vi "SLL DE AI Driver.vi"(7 "AI Driver Option":T2, 8 "error in (no error)":errorcluster, 10 "AI Channel Name Array":T1[](array[typedef]), 11 "AI Channel Name":T1) -> (0 "error out":errorcluster, 2 "AI Channel Value Array":dbl[](array[numeric]), 3 "AI Channel Value":dbl)   [LabVIEW 2009]
doc: "Copyright © 2005, Soliton Technologies.\nAll rights reserved."
uses:
  Controls/SLL DE AI Global Options.ctl
  Controls/SLL DE List of Analog Inputs.ctl
  Controls/SLL DE DAQ Global Elements.ctl
  Controls/SLL DE DAQ Global Options.ctl
  <vilib>/DAQmx/read.llb/DAQmx Read (Analog 1D DBL 1Chan NSamp).vi
  <vilib>/Analysis/NI_AALBase.lvlib
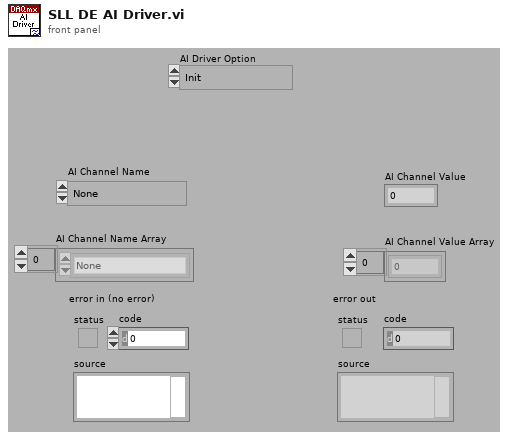
[diagram p1: front panel]
types:
  T1 = typedef "SLL DE List of Analog Inputs.ctl" = enum16{"None"}
  T2 = typedef "SLL DE AI Global Options.ctl" = enum16{"Init", "Write Line", "Write Array", "Read Line", "Read Array", "Read Full Status", "Write Full Status"}
  T3 = typedef "SLL DE DAQ Global Elements.ctl" = enum16{"AI Error", "AO Error", "DI Error", "DO Error", "AI Restart", "DI Restart", "AI Running", "AO Running", "DI Running", "DO Running", "DAQ Exit?"}
  T4 = typedef "SLL DE DAQ Global Options.ctl" = enum16{"Init", "Write 1", "Read 1", "Write Array", "Read Array", "Clear"}
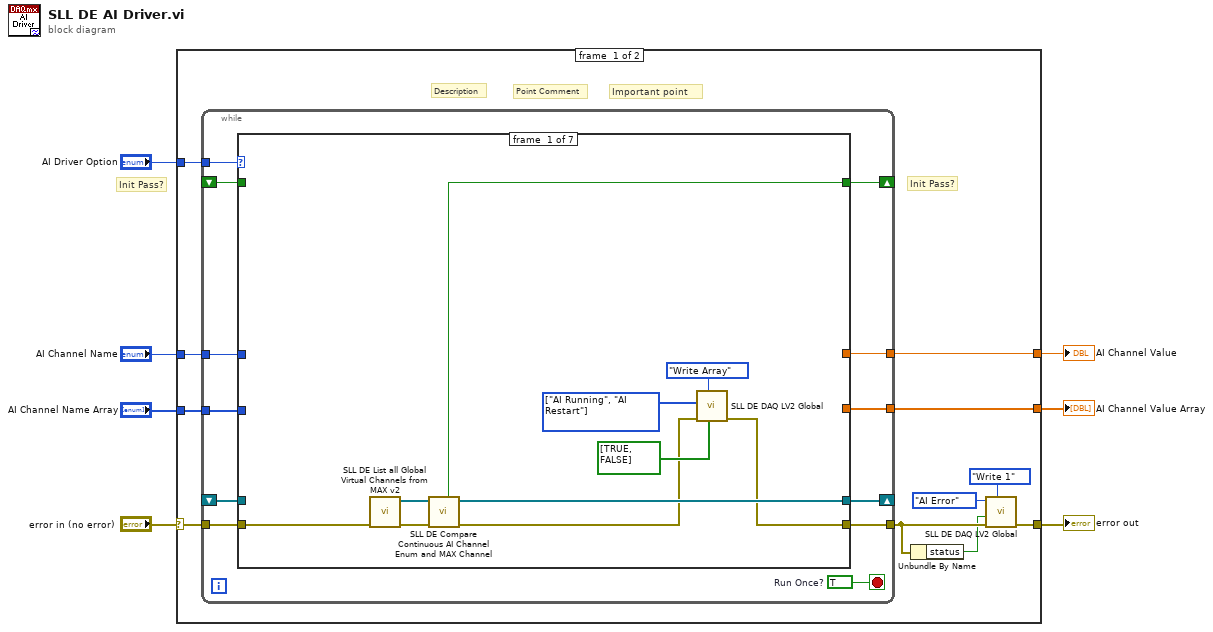
[diagram p0: block diagram]
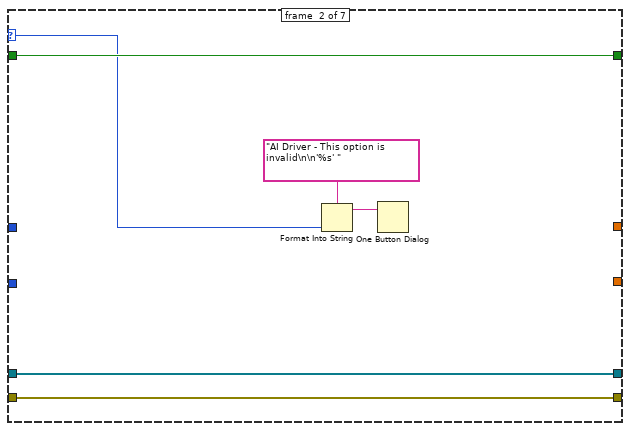
[diagram p2: hidden frame]
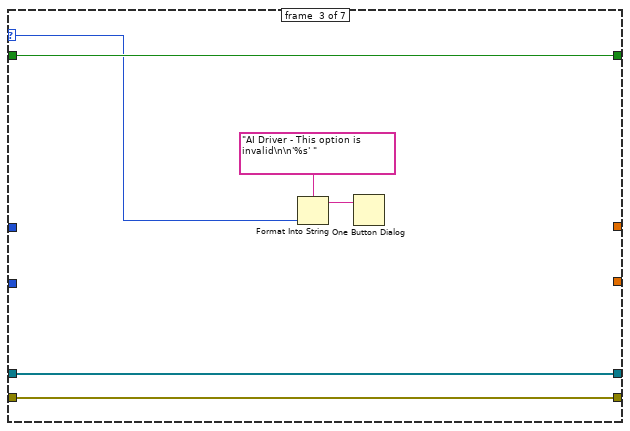
[diagram p3: hidden frame]
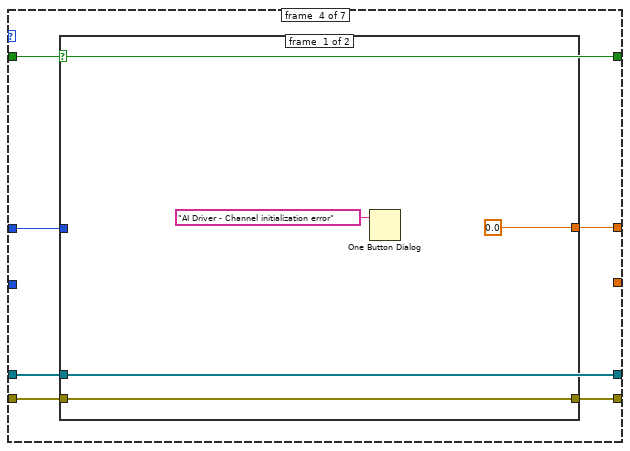
[diagram p4: hidden frame]
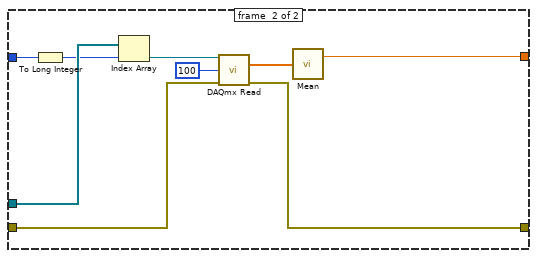
[diagram p5: hidden frame]
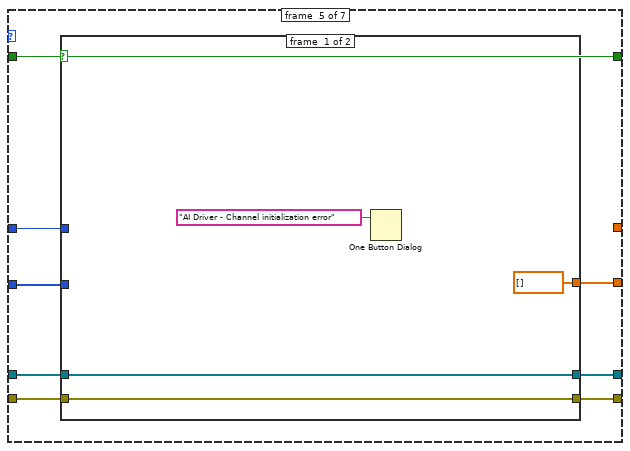
[diagram p6: hidden frame]
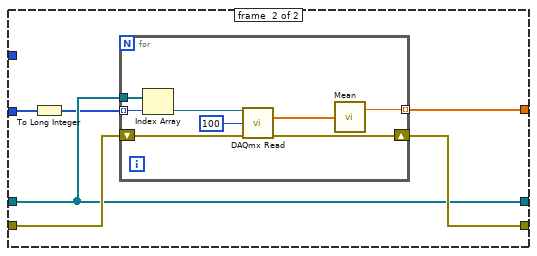
[diagram p7: hidden frame]
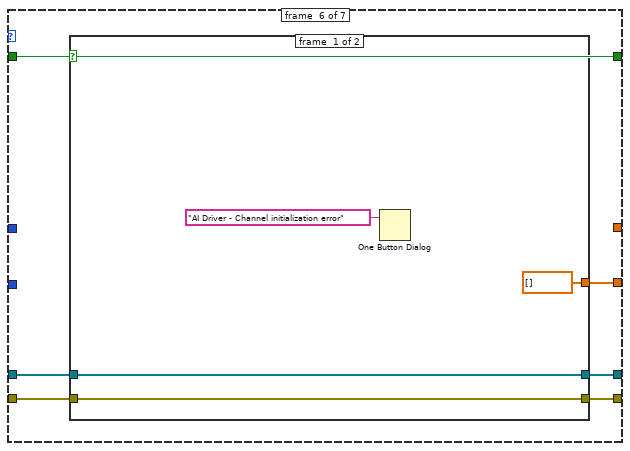
[diagram p8: hidden frame]
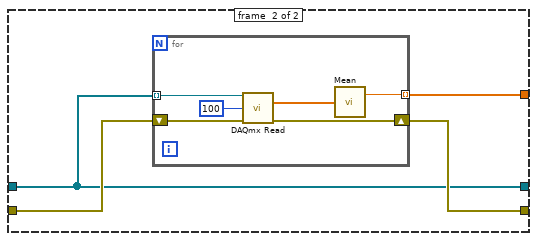
[diagram p9: hidden frame]
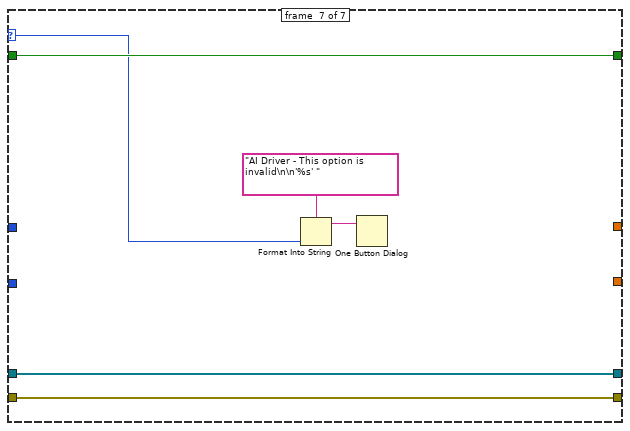
[diagram p10: hidden frame]
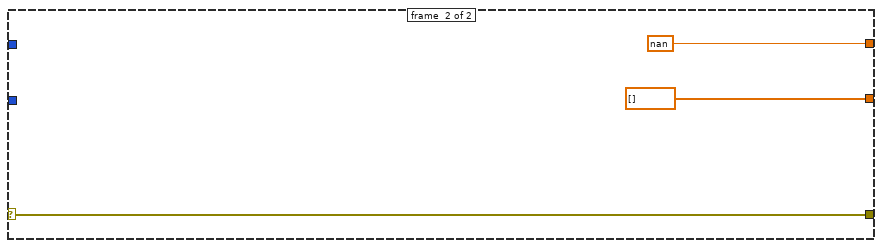
[diagram p11: hidden frame]
diagram:
  # "Init Pass?"
  n1 = case shown="No Error" "error in (no error)" {
    selector: "error in (no error)" -> [w18 w125]
    tunnel: [w11 w125] -> w6
    tunnel: "AI Driver Option" -> [w17 _]
    tunnel: "AI Channel Name" -> [w16 _]
    tunnel: [w15 nan ("mean")] -> w3
    tunnel: "AI Channel Name Array" -> [w14 _]
    tunnel: [w13 dbl[] []] -> w1
    frame #0 {
      # "Init Pass?"
      # "Point Comment"
      # "Important point"
      # "Description"
      n2 = while {
        tunnel: w18 -> [w29]
        tunnel: [w28] -> w9
        shift-right: [w27] -> _
        shift-left: _ -> [w24]
        shift-right: [w26] -> _
        shift-left: _ -> [w23]
        tunnel: w17 -> [w25]
        tunnel: w16 -> [w22]
        tunnel: [w21] -> w15
        tunnel: w14 -> [w20]
        tunnel: [w19] -> w13
        stop <- w30 stop-if-true
        w30 = TRUE  # Run Once?
        n3 = case shown="\"Read Line\"" w25 {
          selector: w25 -> [_ w41 w47 _ _ _ w117]
          tunnel: w29 -> [w38 w44 w50 w56 w78 w102 w121]
          tunnel: [w31 w44 w50 w55 w75 w98 w121] -> w28
          tunnel: [w37 w46 w52 w53 w71 w97 w122] -> w27
          tunnel: [w36 w45 w51 w58 w74 w99 w120] -> w26
          tunnel: w24 -> [_ w46 w52 w53 w71 w97 w122]
          tunnel: w23 -> [_ w45 w51 w58 w77 w101 w120]
          tunnel: w22 -> [_ _ _ w57 w76 _ _]
          tunnel: [_ _ _ w54 _ _ _] -> w21
          tunnel: w20 -> [_ _ _ _ w73 _ _]
          tunnel: [_ _ _ _ w72 w100 _] -> w19
          frame #0 {
            w34 = T3[] [enum."AI Running", enum."AI Restart"] items=["AI Error", "AO Error", "DI Error", "DO Error", "AI Restart", "DI Restart", "AI Running", "AO Running", "DI Running", "DO Running", "DAQ Exit?"] ("Elements Array")
            n4 = call "SLL DE List all Global Virtual Channels from MAX v2.vi"("error in (no error)"=w38) -> ("error out"=w39:errorcluster, "Analog Input"=w40:refnum<k21>[])  [unwired: 4 in, 5 out]
            n5 = call "SLL DE Compare Continuous AI Channel Enum and MAX Channel.vi"("error in (no error)"=w39, "Analog Input Channels"=w40) -> ("error out"=w32:errorcluster, "Channels Out"=w36:refnum<k21>[], "Pass?"=w37:bool)  [unwired: 7 in]
            n6 = call "SLL DE DAQ LV2 Global.vi"("Status Array In"=bool[] [TRUE, FALSE], "Option"=SLL_DE_DAQ_Global_Options."Write Array", "error in (no error)"=w32, "Elements Array"=w34) -> ("error out"=w31:errorcluster)  [unwired: 5 in, 2 out]
          }
          frame #1 {
            n7 = Format Into String(format string="AI Driver - This option is invalid\n\n'%s' " ("message"), w41) -> (resulting string=w42:string)  [unwired: 2 in, 1 out]
            n8 = One Button Dialog(message=w42) -> ()  [unwired: 1 in, 1 out]
          }
          frame #2 {
            n9 = Format Into String(format string="AI Driver - This option is invalid\n\n'%s' " ("message"), w47) -> (resulting string=w48:string)  [unwired: 2 in, 1 out]
            n10 = One Button Dialog(message=w48) -> ()  [unwired: 1 in, 1 out]
          }
          frame #3 {
            n11 = case shown="True" w53 {
              tunnel: w58 -> [_ w68]
              tunnel: w57 -> [_ w67]
              tunnel: w56 -> [w60 w64]
              tunnel: [w60 w63] -> w55
              tunnel: [0.0 ("mean") w62] -> w54
              frame #0 {
                n12 = One Button Dialog(message="AI Driver - Channel initialization error") -> ()  [unwired: 1 in, 1 out]
              }
              frame #1 {
                n13 = To Long Integer(number=w67) -> (32bit integer=w66:i32)
                n14 = Index Array(array=w68, index=w66) -> (element=w65:refnum<k21>)
                n15 = call-poly <vilib>:"DAQmx Read.vi"("task/channels in"=w65, "number of samples per channel"=100, "error in"=w64) -> ("data"=w69:dbl[], "error out"=w63:errorcluster)  [unwired: 10 in, 1 out]
                n16 = call <vilib>:"Mean.vi"("X"=w69) -> ("mean"=w62:dbl)  [unwired: 1 out]
              }
            }
          }
          frame #4 {
            n17 = case shown="True" w71 {
              tunnel: w77 -> [w80 w85]
              tunnel: w76 -> [_ _]
              tunnel: w78 -> [w82 w88]
              tunnel: [w82 w87] -> w75
              tunnel: [dbl[] [] w86] -> w72
              tunnel: [w80 w85] -> w74
              tunnel: w73 -> [_ w84]
              frame #0 {
                n18 = One Button Dialog(message="AI Driver - Channel initialization error") -> ()  [unwired: 1 in, 1 out]
              }
              frame #1 {
                n19 = To Long Integer(number=w84) -> (32bit integer=w83:i32[])
                n20 = for {
                  tunnel: w83 -> [w94] mode=indexing
                  tunnel: [w90] -> w86 mode=indexing
                  tunnel: w85 -> [w89]
                  shift-right: [w91] -> w87
                  shift-left: w88 -> [w92]
                  n21 = Index Array(array=w89, index=w94) -> (element=w93:refnum<k21>)
                  n22 = call-poly <vilib>:"DAQmx Read.vi"("task/channels in"=w93, "number of samples per channel"=100, "error in"=w92) -> ("data"=w95:dbl[], "error out"=w91:errorcluster)  [unwired: 10 in, 1 out]
                  n23 = call <vilib>:"Mean.vi"("X"=w95) -> ("mean"=w90:dbl)  [unwired: 1 out]
                }
              }
            }
          }
          frame #5 {
            n24 = case shown="True" w97 {
              tunnel: w101 -> [w104 w107]
              tunnel: w102 -> [w106 w110]
              tunnel: [w106 w109] -> w98
              tunnel: [dbl[] [] w108] -> w100
              tunnel: [w104 w107] -> w99
              frame #0 {
                n25 = One Button Dialog(message="AI Driver - Channel initialization error") -> ()  [unwired: 1 in, 1 out]
              }
              frame #1 {
                n26 = for {
                  tunnel: [w112] -> w108 mode=indexing
                  tunnel: w107 -> [w111] mode=indexing
                  shift-right: [w113] -> w109
                  shift-left: w110 -> [w114]
                  n27 = call-poly <vilib>:"DAQmx Read.vi"("task/channels in"=w111, "number of samples per channel"=100, "error in"=w114) -> ("data"=w115:dbl[], "error out"=w113:errorcluster)  [unwired: 10 in, 1 out]
                  n28 = call <vilib>:"Mean.vi"("X"=w115) -> ("mean"=w112:dbl)  [unwired: 1 out]
                }
              }
            }
          }
          frame #6 {
            n29 = Format Into String(format string="AI Driver - This option is invalid\n\n'%s' " ("message"), w117) -> (resulting string=w118:string)  [unwired: 2 in, 1 out]
            n30 = One Button Dialog(message=w118) -> ()  [unwired: 1 in, 1 out]
          }
        }
      }
      n31 = Unbundle By Name(w9) -> ("status"=w8:bool)
      n32 = call "SLL DE DAQ LV2 Global.vi"("Option"=SLL_DE_DAQ_Global_Options."Write 1", "error in (no error)"=w9, "Status In"=w8, "Element"=SLL_DE_DAQ_Global_Elements."AI Error") -> ("error out"=w11:errorcluster)  [unwired: 5 in, 2 out]
    }
    frame #1 {
    }
  }
  "error out" <- w6
  "AI Channel Value" <- w3
  "AI Channel Value Array" <- w1
